vi "Create Frame Host LLP Packets.vi"(0 "frame configuration":T1={"pixel data type"=enum."RAW 8", "horizontal resolution"=0, "vertical resolution"=0, "virtual channel"=0.0, "include line sync packets"=FALSE}, 1 "Array":u8[][](array[numeric]), 5 "frame number":u16, 11 "error in (no error)":errorcluster) -> (4 "frame packets":T3[](array[typedef]), 15 "error out":errorcluster)   [LabVIEW 2025, in "GettingStarted_Gen_148X_Host.lvlib"]
uses:
  GettingStarted_Gen_148X_Host.lvlib
  <instrlib>/FlexRIO/CSI-2/v2/Host/Types/Host LLP Packet.ctl
  <instrlib>/FlexRIO/CSI-2/v2/FPGA/Types/LLP Packet Header.ctl
  <instrlib>/FlexRIO/CSI-2/v2/FPGA/Types/LLP Packet Footer.ctl
  Types/Frame Data Configuration.ctl
  <instrlib>/FlexRIO/CSI-2/v2/Common/Types/LLP Data Type.ctl
  <instrlib>/FlexRIO/CSI-2/v2/FPGA/NI CSI-2 API FPGA v2.lvlib
  <instrlib>/FlexRIO/CSI-2/v2/Host/NI CSI-2 API Host v2.lvlib
  <instrlib>/FlexRIO/CSI-2/v2/Common/NI CSI-2 API Common v2.lvlib
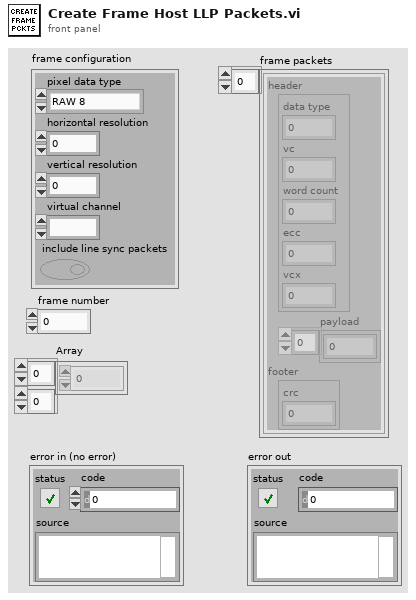
[diagram p1: front panel]
types:
  T1 = typedef "GettingStarted_Gen_148X_Host.lvlib/Frame Data Configuration.ctl" = cluster{"pixel data type":T2, "horizontal resolution":u16, "vertical resolution":u16, "virtual channel":fxp<+,4,4>, "include line sync packets":bool}
  T2 = typedef "NI CSI-2 API Common v2.lvlib/LLP Data Type.ctl" = enum8{"Frame Start", "Frame End", "Line Start", "Line End", "End of Transmission", "Reserved 0", "Reserved 1", "Reserved 2", "Generic Short Packet 1", "Generic Short Packet 2", "Generic Short Packet 3", "Generic Short Packet 4", "Generic Short Packet 5", "Generic Short Packet 6", "Generic Short Packet 7", "Generic Short Packet 8", "Null", "Blanking Data", "Embedded 8-bit non Image Data", "Generic Long Packet 1", "Generic Long Packet 2", "Generic Long Packet 3", "Generic Long Packet 4", "Reserved 3", "YUV420 8-bit", "YUV420 10-bit", "Legacy YUV420 8-bit", "Reserved 4", "YUV420 8-bit Chroma Shifted", "YUV420 10-bit Chroma Shifted", "YUV422 8-bit", "YUV422 10-bit", "RGB444", "RGB555", "RGB565", "RGB666", "RGB888", "Reserved 5", "Reserved 6", "RAW 24", "RAW 6", "RAW 7", "RAW 8", "RAW 10", "RAW 12", "RAW 14", "RAW 16", "RAW 20", "User Defined 8-bit Data 1", "User Defined 8-bit Data 2", "User Defined 8-bit Data 3", "User Defined 8-bit Data 4", "User Defined 8-bit Data 5", "User Defined 8-bit Data 6", "User Defined 8-bit Data 7", "User Defined 8-bit Data 8", "USL Command", "Reserved 7", "Reserved 8", "Reserved 9", "Reserved 10", "Reserved 11", "Reserved 12", "LRTE EPD Spacer"}
  T3 = typedef "NI CSI-2 API Host v2.lvlib/Host LLP Packet.ctl" = cluster{"header":T4, "payload":u8[], "footer":T5}
  T4 = typedef "NI CSI-2 API FPGA v2.lvlib/LLP Packet Header.ctl" = cluster{"word count":u16, "ecc":fxp<+,6,6>, "vcx":fxp<+,2,2>, "data type":fxp<+,6,6>, "vc":fxp<+,2,2>}
  T5 = typedef "NI CSI-2 API FPGA v2.lvlib/LLP Packet Footer.ctl" = cluster{"crc":u16}
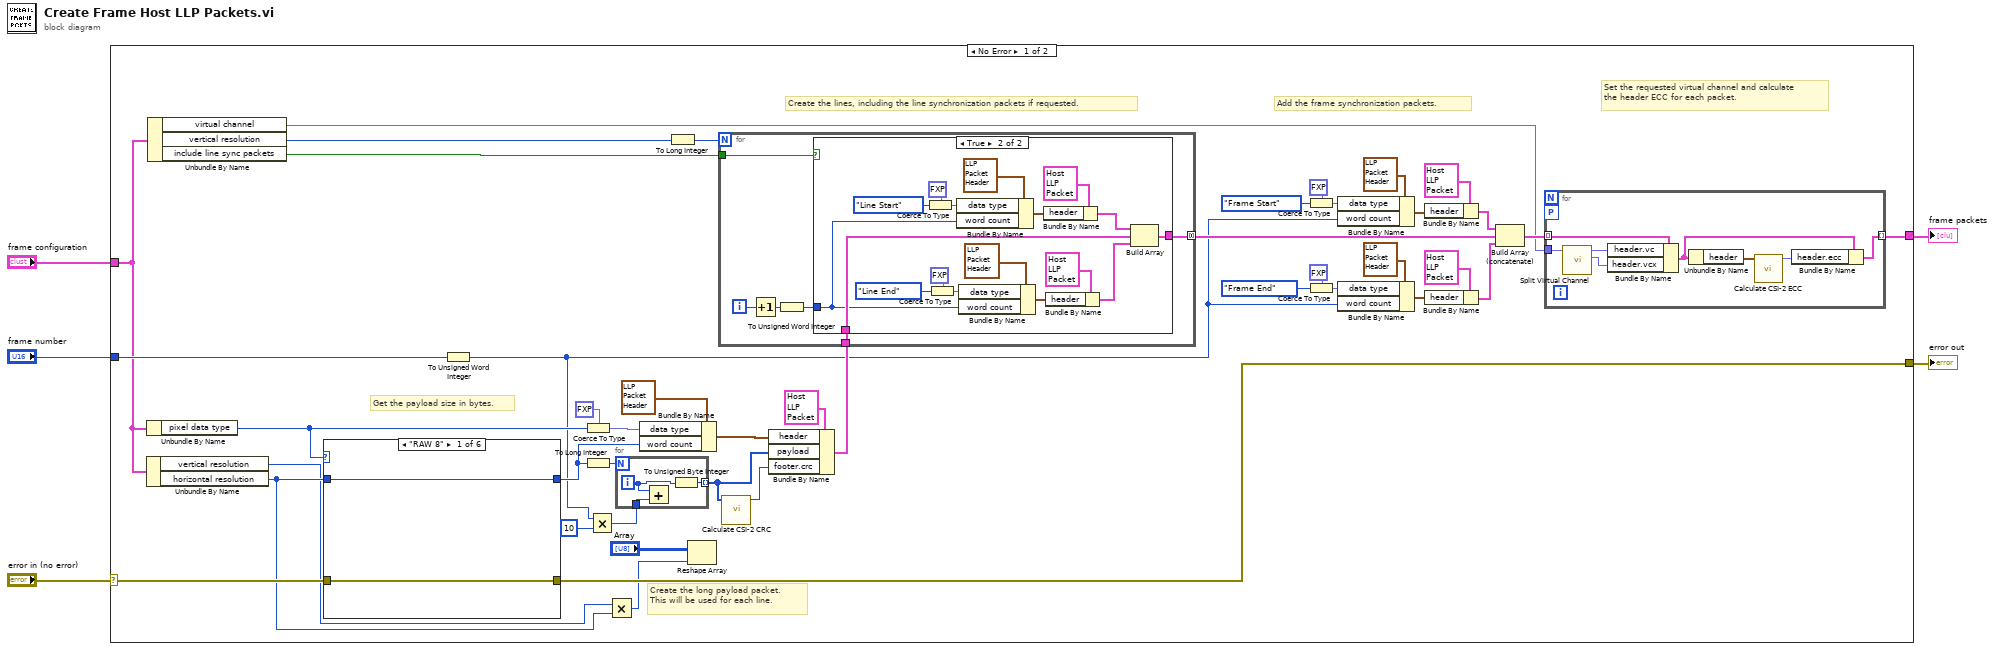
[diagram p0: block diagram]
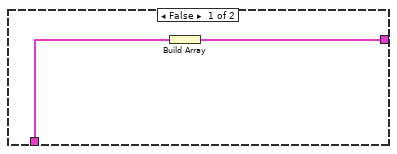
[diagram p2: hidden frame]
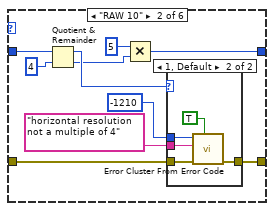
[diagram p3: hidden frame]
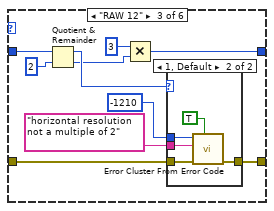
[diagram p5: hidden frame]
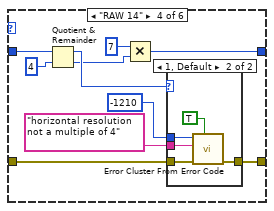
[diagram p7: hidden frame]
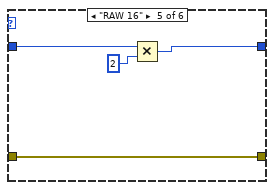
[diagram p9: hidden frame]
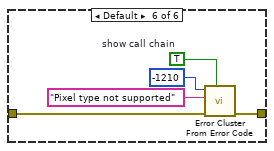
[diagram p10: hidden frame]
diagram:
  n1 = case shown="No Error" "error in (no error)" {
    selector: "error in (no error)" -> [w16 w144]
    tunnel: [w38 _] -> w5
    tunnel: [w48 w144] -> w3
    tunnel: "frame number" -> [w21 _]
    tunnel: "frame configuration" -> [w17 _]
    frame No Error {
      # "Set the requested virtual channel and calculate the header ECC for each packet."
      # "Add the frame synchronization packets."
      # "Create the lines, including the line synchronization packets if requested."
      # "Create the long payload packet.  This will be used for each line."
      # "Get the payload size in bytes."
      n2 = Unbundle By Name(w17) -> ("vertical resolution"=w8:u16, "horizontal resolution"=w9:u16)
      n3 = Unbundle By Name(w17) -> ("pixel data type"=w20:T2)
      n4 = Unbundle By Name(w17) -> ("virtual channel"=w18:fxp<+,4,4>, "vertical resolution"=w19:u16, "include line sync packets"=w15:bool)
      n5 = case shown="\"RAW 8\"" w20 {
        tunnel: w9 -> [w83 w86 w102 w118 w135 _]
        tunnel: [w83 w85 w101 w117 w133 _] -> w42
        tunnel: w16 -> [w82 w93 w109 w125 w132 w139]
        tunnel: [w82 w90 w106 w122 w132 w138] -> w48
        frame "RAW 8" {
        }
        frame "RAW 10" {
          n6 = Quotient & Remainder(x=w86, y=u16 4) -> (x-y*floor(x/y)=w88:u16, floor(x/y)=w84:u16)
          n7 = Multiply(x=u16 5 ("y"), y=w84) -> (x*y=w85:u16)
          n8 = case shown="1, Default" w88 {
            tunnel: w93 -> [w94 w96]
            tunnel: -1210 ("code") -> [_ w98]
            tunnel: "horizontal resolution not a multiple of 4" ("source") -> [_ w97]
            tunnel: [w94 w95] -> w90
            frame 0 {
            }
            frame 1, Default {
              n9 = call <vilib>:"Error Cluster From Error Code.vi"("show call chain? (False)"=TRUE ("show call chain"), "error in (no error)"=w96, "error message (\"\")"=w97, "error code (0)"=w98) -> ("error out"=w95:errorcluster)  [unwired: 5 in]
            }
          }
        }
        frame "RAW 12" {
          n10 = Quotient & Remainder(x=w102, y=u16 2) -> (x-y*floor(x/y)=w104:u16, floor(x/y)=w100:u16)
          n11 = Multiply(x=u16 3 ("y"), y=w100) -> (x*y=w101:u16)
          n12 = case shown="1, Default" w104 {
            tunnel: w109 -> [w110 w112]
            tunnel: -1210 ("code") -> [_ w114]
            tunnel: "horizontal resolution not a multiple of 2" ("source") -> [_ w113]
            tunnel: [w110 w111] -> w106
            frame 0 {
            }
            frame 1, Default {
              n13 = call <vilib>:"Error Cluster From Error Code.vi"("show call chain? (False)"=TRUE ("show call chain"), "error in (no error)"=w112, "error message (\"\")"=w113, "error code (0)"=w114) -> ("error out"=w111:errorcluster)  [unwired: 5 in]
            }
          }
        }
        frame "RAW 14" {
          n14 = Quotient & Remainder(x=w118, y=u16 4) -> (x-y*floor(x/y)=w120:u16, floor(x/y)=w116:u16)
          n15 = Multiply(x=u16 7 ("y"), y=w116) -> (x*y=w117:u16)
          n16 = case shown="1, Default" w120 {
            tunnel: w125 -> [w126 w128]
            tunnel: -1210 ("code") -> [_ w130]
            tunnel: "horizontal resolution not a multiple of 4" ("source") -> [_ w129]
            tunnel: [w126 w127] -> w122
            frame 0 {
            }
            frame 1, Default {
              n17 = call <vilib>:"Error Cluster From Error Code.vi"("show call chain? (False)"=TRUE ("show call chain"), "error in (no error)"=w128, "error message (\"\")"=w129, "error code (0)"=w130) -> ("error out"=w127:errorcluster)  [unwired: 5 in]
            }
          }
        }
        frame "RAW 16" {
          n18 = Multiply(x=w135, y=u16 2) -> (x*y=w133:u16)
        }
        frame Default {
          w140 = TRUE  # show call chain
          n19 = call <vilib>:"Error Cluster From Error Code.vi"("show call chain? (False)"=w140, "error in (no error)"=w139, "error message (\"\")"="Pixel type not supported" ("source"), "error code (0)"=-1210 ("code")) -> ("error out"=w138:errorcluster)  [unwired: 5 in]
        }
      }
      n20 = To Unsigned Word Integer(number=w21) -> (unsigned 16bit integer=w13:u16)
      n21 = Coerce To Type(0:w20, 1:fxp<+,6,6> 0.0 ("data type")) -> (2:w45:fxp<+,6,6>)
      n22 = To Long Integer(number=w42) -> (32bit integer=w47:i32)
      n23 = Multiply(x=w13, y=u16 10) -> (x*y=w12:u16)
      n24 = Multiply(x=w8, y=w9) -> (x*y=w7:u16)
      n25 = for {
        N: w47 -> [_]
        tunnel: [w143] -> w6 mode=indexing
        tunnel: w12 -> [w142]
        i -> [w141]
        n26 = Add(x=w141, y=w142) -> ()  [unwired: 1 out]
        n27 = To Unsigned Byte Integer(number=w141) -> (unsigned 8bit integer=w143:u8)
      }
      n28 = Bundle By Name(cluster=T4 {"word count"=0, "ecc"=0.0, "vcx"=0.0, "data type"=0.0, "vc"=0.0} ("header"), "data type"=w45, "word count"=w42) -> (w46:T4)
      n29 = To Long Integer(number=w19) -> (32bit integer=w22:i32)
      n30 = Reshape Array("Array", w7) -> ()  [unwired: 1 out]
      n31 = call <instrlib>:"Calculate CSI-2 CRC.vi"("payload"=w6) -> ("crc"=w41:u16)  [unwired: 10 in]
      n32 = Bundle By Name(cluster=T3 {"header"={"word count"=0, "ecc"=0.0, "vcx"=0.0, "data type"=0.0, "vc"=0.0}, "payload"=[], "footer"={"crc"=0}}, "header"=w46, "payload"=w6, "footer.crc"=w41) -> (w14:T3)
      n33 = for {
        N: w22 -> [_]
        tunnel: w15 -> [w50]
        tunnel: w14 -> [w51]
        tunnel: [w49] -> w25 mode=concatenating
        i -> [w52]
        n34 = Increment(x=w52) -> (x+1=w54:i32)
        n35 = To Unsigned Word Integer(number=w54) -> (unsigned 16bit integer=w53:u16)
        n36 = case shown="True" w50 {
          tunnel: w53 -> [_ w58]
          tunnel: w51 -> [w56 w60]
          tunnel: [w55 w57] -> w49
          frame False {
            n37 = Build Array(w56) -> (w55:T3[])
          }
          frame True {
            n38 = Coerce To Type(0:LLP_Data_Type."Line Start" ("Enum"), 1:fxp<+,6,6> 0.0 ("data type")) -> (2:w69:fxp<+,6,6>)
            n39 = Coerce To Type(0:LLP_Data_Type."Line End" ("Enum"), 1:fxp<+,6,6> 0.0 ("data type")) -> (2:w63:fxp<+,6,6>)
            n40 = Bundle By Name(cluster=T4 {"word count"=0, "ecc"=0.0, "vcx"=0.0, "data type"=0.0, "vc"=0.0} ("header"), "data type"=w69, "word count"=w58) -> (w72:T4)
            n41 = Bundle By Name(cluster=T4 {"word count"=0, "ecc"=0.0, "vcx"=0.0, "data type"=0.0, "vc"=0.0} ("header"), "data type"=w63, "word count"=w58) -> (w66:T4)
            n42 = Bundle By Name(cluster=T3 {"header"={"word count"=0, "ecc"=0.0, "vcx"=0.0, "data type"=0.0, "vc"=0.0}, "payload"=[], "footer"={"crc"=0}}, "header"=w72) -> (w61:T3)
            n43 = Bundle By Name(cluster=T3 {"header"={"word count"=0, "ecc"=0.0, "vcx"=0.0, "data type"=0.0, "vc"=0.0}, "payload"=[], "footer"={"crc"=0}}, "header"=w66) -> (w59:T3)
            n44 = Build Array(w61, w60, w59) -> (w57:T3[])
          }
        }
      }
      n45 = Coerce To Type(0:LLP_Data_Type."Frame Start" ("Enum"), 1:fxp<+,6,6> 0.0 ("data type")) -> (2:w31:fxp<+,6,6>)
      n46 = Coerce To Type(0:LLP_Data_Type."Frame End" ("Enum"), 1:fxp<+,6,6> 0.0 ("data type")) -> (2:w32:fxp<+,6,6>)
      n47 = Bundle By Name(cluster=T4 {"word count"=0, "ecc"=0.0, "vcx"=0.0, "data type"=0.0, "vc"=0.0} ("header"), "data type"=w31, "word count"=w13) -> (w28:T4)
      n48 = Bundle By Name(cluster=T4 {"word count"=0, "ecc"=0.0, "vcx"=0.0, "data type"=0.0, "vc"=0.0} ("header"), "data type"=w32, "word count"=w13) -> (w35:T4)
      n49 = Bundle By Name(cluster=T3 {"header"={"word count"=0, "ecc"=0.0, "vcx"=0.0, "data type"=0.0, "vc"=0.0}, "payload"=[], "footer"={"crc"=0}}, "header"=w28) -> (w24:T3)
      n50 = Bundle By Name(cluster=T3 {"header"={"word count"=0, "ecc"=0.0, "vcx"=0.0, "data type"=0.0, "vc"=0.0}, "payload"=[], "footer"={"crc"=0}}, "header"=w35) -> (w23:T3)
      n51 = Build Array (concatenate)(w24, w25, w23) -> (w39:T3[])
      n52 = for {
        tunnel: w39 -> [w81] mode=indexing
        tunnel: w18 -> [w78]
        tunnel: [w74] -> w38 mode=indexing
        workers-P: _ -> [_]
        n53 = call <instrlib>:"Split Virtual Channel.vi"("virtual channel"=w78) -> ("vcx"=w79:fxp<+,2,2>, "vc"=w80:fxp<+,2,2>)  [unwired: 9 in]
        n54 = Bundle By Name(cluster=w81, "header.vc"=w80, "header.vcx"=w79) -> (w75:T3)
        n55 = Unbundle By Name(w75) -> ("header"=w77:T4)
        n56 = call <instrlib>:"Calculate CSI-2 ECC.vi"("header"=w77) -> ("ecc"=w76:fxp<+,6,6>)  [unwired: 10 in]
        n57 = Bundle By Name(cluster=w75, "header.ecc"=w76) -> (w74:T3)
      }
    }
    frame Error {
    }
  }
  "error out" <- w3
  "frame packets" <- w5
